vi "State Entry.vi"(8 "error in (no error)":errorcluster, 11 "View Model":T1) -> (0 "error out":errorcluster, 3 "View Model":T1)   [LabVIEW 2013]
doc: "Initializes state information at beginning of transition."
uses:
  View Model/Controls/View Model.ctl
  Error/Controls/Error Model.ctl
  Error/Controls/Error Types.ctl
  View Model/Controls/Shared Model.ctl
  Controls/Elevator Model.ctl
  Controls/Controller Overhead.ctl
  Controls/Elevator States.ctl
  Controls/Elevator Location.ctl
  Controls/Elevator Command Event.ctl
  Controls/Elevator Commands.ctl
  Configuration/Controls/Configuration Model.ctl
  Configuration/Controls/Configuration Data.ctl
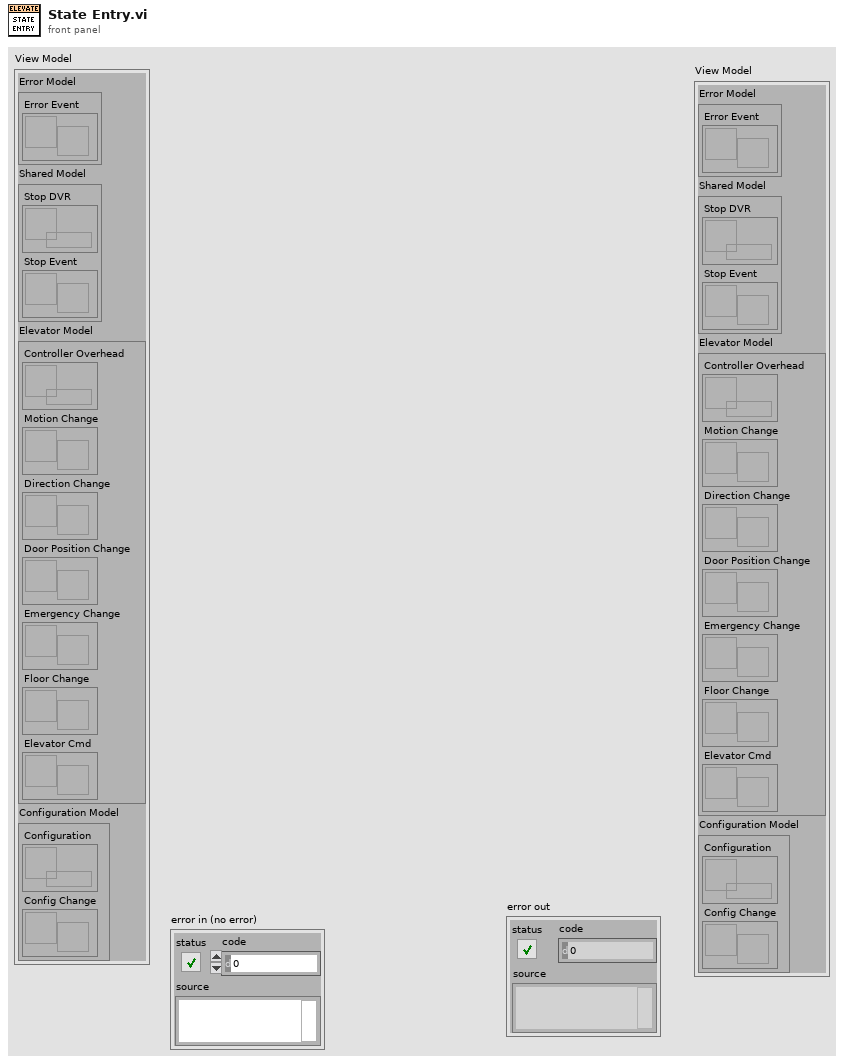
[diagram p1: front panel]
types:
  T1 = typedef "View Model.ctl" = cluster{"Error Model":T2, "Shared Model":T3, "Elevator Model":T4, "Configuration Model":T5}
  T2 = typedef "Error Model.ctl" = cluster{"Error Event":refnum<user-event>}
  T3 = typedef "Shared Model.ctl" = cluster{"Stop DVR":refnum<data-value>, "Stop Event":refnum<user-event>}
  T4 = typedef "Elevator Model.ctl" = cluster{"Controller Overhead":refnum<data-value>, "Motion Change":refnum<user-event>, "Direction Change":refnum<user-event>, "Door Position Change":refnum<user-event>, "Emergency Change":refnum<user-event>, "Floor Change":refnum<user-event>, "Elevator Cmd":refnum<user-event>}
  T5 = typedef "Configuration Model.ctl" = cluster{"Configuration":refnum<data-value>, "Config Change":refnum<user-event>}
  T6 = typedef "Elevator States.ctl" = enum16{"Initial State", "Open Doors", "Close Doors", "Start Move", "Move", "Finish Move", "Emergency", "Analysis"}
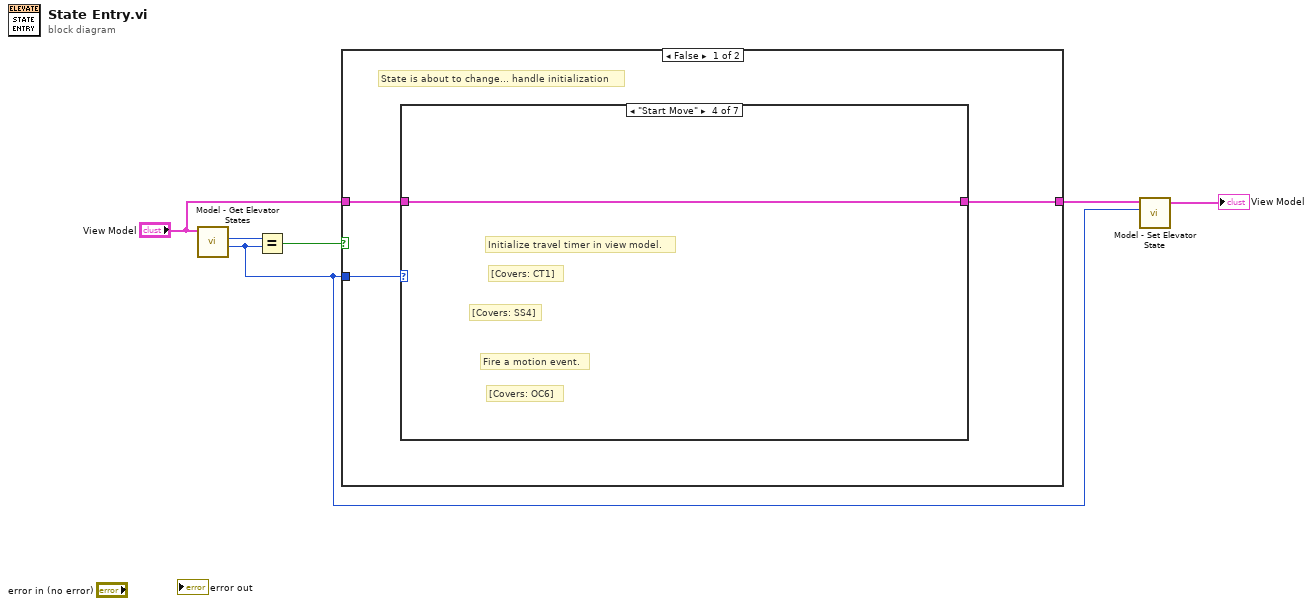
[diagram p0: block diagram]
diagram:
  n1 = call "Model - Get Elevator States.vi"("View Model"="View Model") -> ("Next Elevator State"=w2:T6, "Elevator State"=w5:T6)  [unwired: 7 in, 2 out]
  n2 = Equal?(x=w5, y=w2) -> (x = y?=w6:bool)
  n3 = case shown="False" w6 {
    tunnel: w2 -> [w9 _]
    tunnel: "View Model" -> [w8 w17]
    tunnel: [w7 w17] -> w3
    frame False {
      # "State is about to change... handle initialization"
      n4 = case shown="\"Start Move\"" w9 {
        tunnel: w8 -> [w10 w11 w12 w13 w14 w15 w16]
        tunnel: [w10 w11 w12 w13 w14 w15 w16] -> w7
        frame "Initial State", Default {
        }
        frame "Open Doors" {
          # "[Covers: OC3A]"
          # "[Covers: OC3]"
          # "Start open door timer"
        }
        frame "Close Doors" {
        }
        frame "Start Move" {
          # "[Covers: OC6]"
          # "Fire a motion event."
          # "[Covers: CT1]"
          # "[Covers: SS4]"
          # "Initialize travel timer in view model."
        }
        frame "Emergency" {
        }
        frame "Move" {
        }
        frame "Finish Move" {
        }
      }
    }
    frame True {
    }
  }
  n5 = call "Model - Set Elevator State.vi"("Elevator State"=w2, "View Model"=w3) -> ("View Model"=→"View Model":T1)  [unwired: 8 in, 1 out]
